vi "gl_Pockels control globals.vi"() -> ()   [LabVIEW 2013]
panel:
  in  "Pockels \"Low\" time (us)":dbl=20.0
  in  "Standby Laser Power (%)":dbl=5.0 format="%#_13g"
  in  "Pockels mod previous state":bool=TRUE
  in  "Pockels voltage max":dbl=2.0 format="%#_13g"
  in  "Pockels voltage min":dbl format="%#_13g"
  in  "Funct. acq. pockels modulation?":bool=TRUE
  # "<---- Pockels modulation enabled only in functional acquisition"
  # "<--- at modulation stop and before z-stacks and functional acquisition"
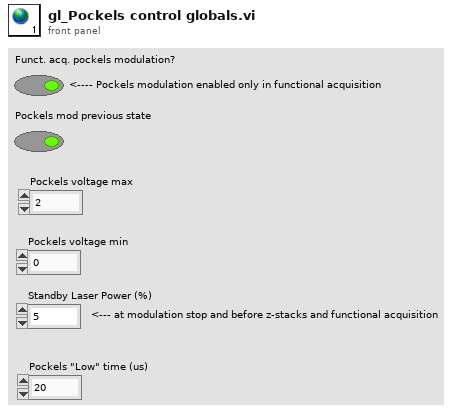
[diagram p1: front panel]
diagram:
